vi "setPosition.vi"(6 "Delay between send and receive [ms]":i32=100, 8 "error in (no error)":errorcluster, 10 "wavelength":dbl format="%#_13g", 11 "Monochromator in":refnum<class "Monochromator.lvclass">) -> (0 "error out":errorcluster, 1 "ID":i32, 2 "results-JSON string":string, 3 "Monochromator out":refnum<class "Monochromator.lvclass">)   [LabVIEW 2023, in "Monochromator.lvclass"]
uses:
  Monochromator.lvclass
  Monochromator.lvclass/Monochromator.ctl
  7fe8abea-6ecd-46de-aa11-ce8637911b6a.vi
  GenericDevice/GenericDevice.lvclass
  <vilib>/IlluminatedG/lv-web-crypto/lv-json/JSON/JSON.lvlib
  35d46a5a-fd7c-4445-96f4-e877dae8f93b.vi
panel:
  # "Connector Pane"
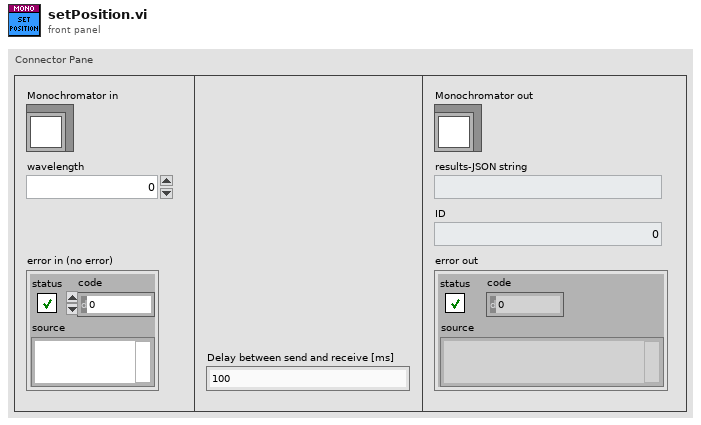
[diagram p1: front panel]
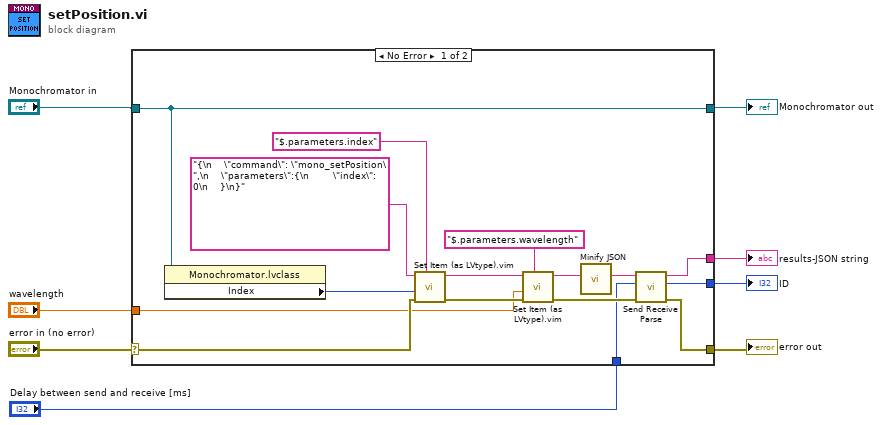
[diagram p0: block diagram]
diagram:
  n1 = case shown="No Error" "error in (no error)" {
    selector: "error in (no error)" -> [w20 w26]
    tunnel: [w17 w26] -> w5
    tunnel: [w22 w25] -> w7
    tunnel: "Monochromator in" -> [w22 w25]
    tunnel: [w19 _] -> w3
    tunnel: [w18 _] -> w4
    tunnel: "wavelength" -> [w10 _]
    tunnel: "Delay between send and receive [ms]" -> [w9 _]
    frame No Error {
      n2 = property class="Monochromator.lvclass"(reference=w22) -> ("Index"=w21:i32)  [unwired: 1 in, 2 out]
      n3 = call "Set Item (as LVtype).vim"("$Path or Item Name"="$.parameters.index", "error in (no error)"=w20, "Anything"=w21, "JSON"="{\n    \"command\": \"mono_setPosition\",\n    \"parameters\":{\n        \"index\": 0\n    }\n}") -> ("error out"=w14:errorcluster, "<JSON>"=w12:string)  [unwired: 4 in, 1 out]
      n4 = call "Set Item (as LVtype).vim"("$Path or Item Name"="$.parameters.wavelength", "error in (no error)"=w14, "Anything"=w10, "JSON"=w12) -> ("error out"=w13:errorcluster, "<JSON>"=w11:string)  [unwired: 4 in, 1 out]
      n5 = call <vilib>:"Minify JSON.vi"("JSON String"=w11) -> ("Minified JSON"=w16:string)  [unwired: 10 in]
      n6 = call "Send Receive Parse.vi"("error in"=w13, "Delay between send and receive [ms]"=w9, "<JSON>"=w16) -> ("error out"=w17:errorcluster, "ID"=w18:i32, "results-JSON string"=w19:string)  [unwired: 6 in]
    }
    frame Error {
    }
  }
  "error out" <- w5
  "Monochromator out" <- w7
  "ID" <- w4
  "results-JSON string" <- w3
